vi "LVClass_WavefrontCorrectorSet Get WavefrontCorrectorParameter.vi"(0 "WavefrontCorrectorSet in":refnum<class "WavefrontCorrectorSet.lvclass">, 11 "error in (no error)":errorcluster) -> (4 "WavefrontCorrectorSet out":refnum<class "WavefrontCorrectorSet.lvclass">, 6 "AllCurrentValueSetAndGet":T1[](array[typedef]), 8 "AllCurrentValueGet":T1[](array[typedef]), 15 "error out":errorcluster)   [LabVIEW 2020, in "WavefrontCorrectorSet.lvclass"]
doc: "WavefrontCorrector parameter name getter given its position in the parameters\nlist.\n\n--------------------------------------------------------------------------------\n\n<B>wavefrontcorrector_setIn </B> : WavefrontCorrectorSet object.\n<B>wavefrontcorrector_setOut </B> : WavefrontCorrectorSet object.\n<B>index </B> : Parameter index.\n<B>parameter_name </B> : Parameter name.\n<B>ErrorIn </B> : Error\n<B>ErrorOut </B> : Error\n\n--------------------------------------------------------------------------------"
uses:
  WavefrontCorrectorSet.lvclass
  CameraParametersSetup.ctl
  CameraParameters_Type.ctl
  WavefrontCorrectorSet.lvclass/WavefrontCorrectorSet.ctl
  LVClass_WavefrontCorrectorSet Read AllValueSetAndGet.vi
  LVClass_WavefrontCorrectorSet Read AllValueGet.vi
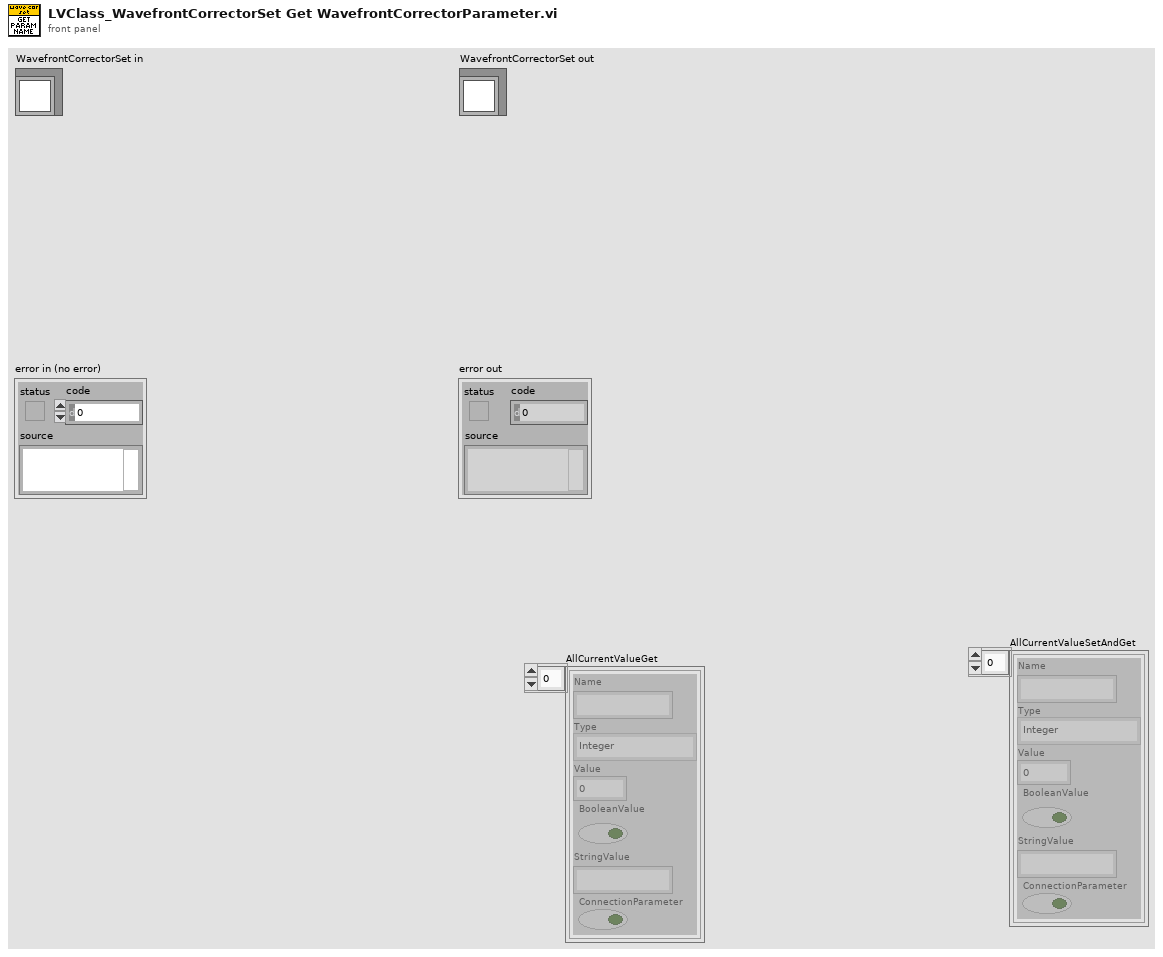
[diagram p1: front panel]
types:
  T1 = typedef "CameraParametersSetup.ctl" = cluster{"Name":string, "Type":T2, "Value":dbl, "BooleanValue":bool, "StringValue":string, "ConnectionParameter":bool}
  T2 = typedef "CameraParameters_Type.ctl" = enum16{"Integer", "Real", "String", "Boolean"}
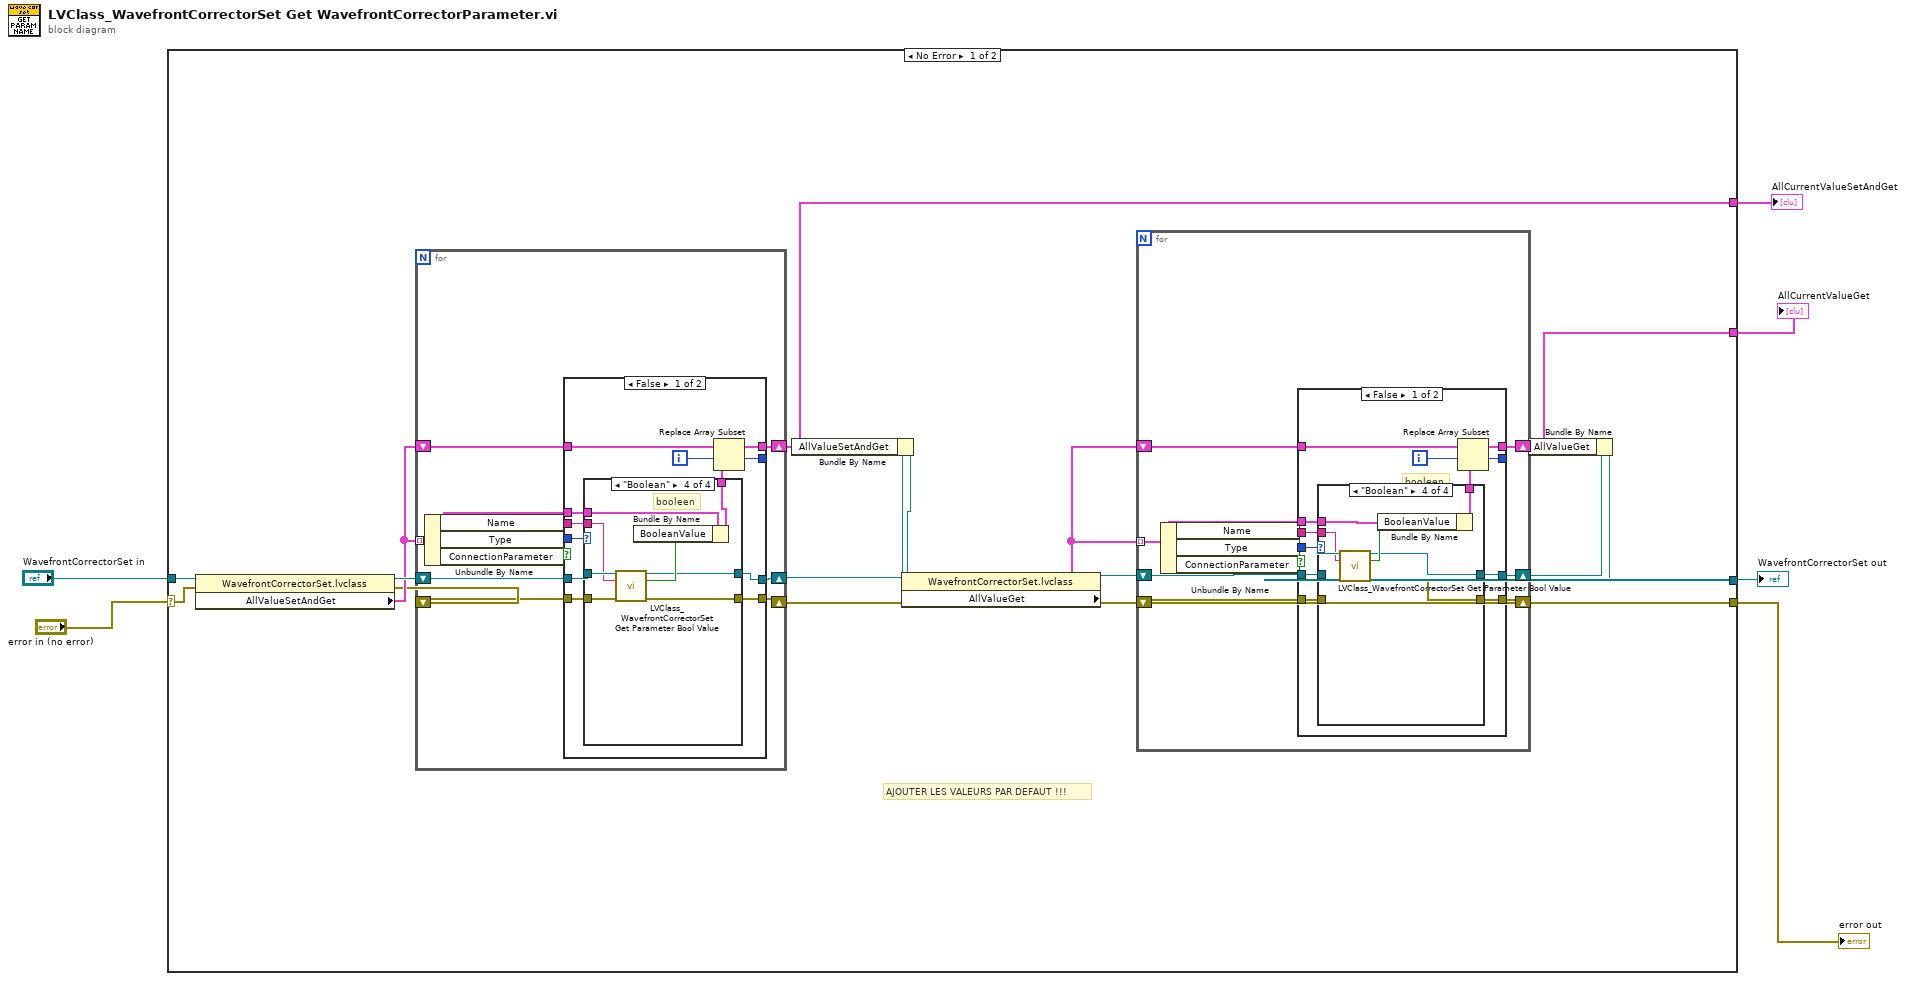
[diagram p0: block diagram]
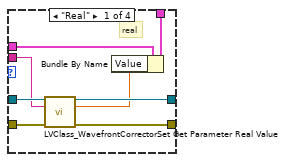
[diagram p2: hidden frame]
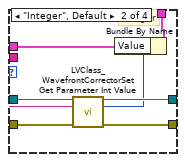
[diagram p3: hidden frame]
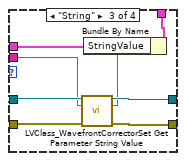
[diagram p4: hidden frame]
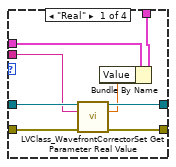
[diagram p6: hidden frame]
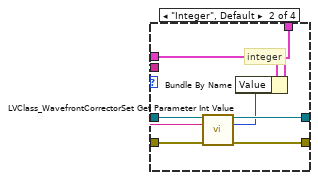
[diagram p7: hidden frame]
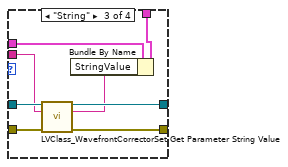
[diagram p8: hidden frame]
diagram:
  n1 = case shown="No Error" "error in (no error)" {
    selector: "error in (no error)" -> [w8 w136]
    tunnel: "WavefrontCorrectorSet in" -> [w11 w137]
    tunnel: [w10 w137] -> w4
    tunnel: [w12 _] -> w2
    tunnel: [w9 w136] -> w3
    tunnel: [w7 _] -> w1
    frame No Error {
      # "AJOUTER LES VALEURS PAR DEFAUT !!!"
      n2 = property class="WavefrontCorrectorSet.lvclass"(reference=w11, error in=w8) -> (reference out=w20:refnum<class "WavefrontCorrectorSet.lvclass">, error out=w18:errorcluster, "AllValueSetAndGet"=w19:T1[])
      n3 = for {
        shift-right: [w89] -> w15
        shift-left: w18 -> [w82]
        shift-right: [w88] -> w21
        shift-left: w20 -> [w83]
        shift-right: [w86] -> w12
        shift-left: w19 -> [w87]
        tunnel: w19 -> [w80] mode=indexing
        i -> [w85]
        n4 = Unbundle By Name(w80) -> ("Name"=w84:string, "Type"=w81:T2, "ConnectionParameter"=w79:bool)
        n5 = case shown="False" w79 {
          tunnel: [w100 w133] -> w89
          tunnel: [w99 w134] -> w88
          tunnel: w87 -> [w98 w135]
          tunnel: [w97 w135] -> w86
          tunnel: w85 -> [w96 _]
          tunnel: w84 -> [w94 _]
          tunnel: w83 -> [w93 w134]
          tunnel: w82 -> [w92 w133]
          tunnel: w81 -> [w91 _]
          tunnel: w80 -> [w90 _]
          frame False {
            n6 = case shown="\"Boolean\"" w91 {
              tunnel: w90 -> [w102 w109 w118 w131]
              tunnel: w94 -> [w106 w114 w120 w128]
              tunnel: [w105 w113 w122 w126] -> w100
              tunnel: w93 -> [w108 w116 w124 w130]
              tunnel: w92 -> [w107 w115 w121 w129]
              tunnel: [w104 w112 w123 w127] -> w99
              tunnel: [w103 w111 w117 w125] -> w95
              frame "Real" {
                n7 = call "LVClass_WavefrontCorrectorSet Get Parameter Real Value.vi"("WavefrontCorrectorSet in"=w108, "parameter_name"=w106, "error in (no error)"=w107) -> ("WavefrontCorrectorSet out"=w104:refnum<class "WavefrontCorrectorSet.lvclass">, "Value"=w101:dbl, "error out"=w105:errorcluster)  [unwired: 10 in]
                n8 = Bundle By Name(cluster=w102, "Value"=w101) -> (w103:T1)
              }
              frame "Integer", Default {
                # "integer"
                n9 = call "LVClass_WavefrontCorrectorSet Get Parameter Int Value.vi"("WavefrontCorrectorSet in"=w116, "parameter_name"=w114, "error in (no error)"=w115) -> ("WavefrontCorrectorSet out"=w112:refnum<class "WavefrontCorrectorSet.lvclass">, "Value"=w110:i32, "error out"=w113:errorcluster)  [unwired: 10 in]
                n10 = Bundle By Name(cluster=w109, "Value"=w110) -> (w111:T1)
              }
              frame "String" {
                n11 = call "LVClass_WavefrontCorrectorSet Get Parameter String Value.vi"("WavefrontCorrectorSet in"=w124, "parameter name"=w120, "error in (no error)"=w121) -> ("WavefrontCorrectorSet out"=w123:refnum<class "WavefrontCorrectorSet.lvclass">, "Value"=w119:string, "error out"=w122:errorcluster)  [unwired: 10 in]
                n12 = Bundle By Name(cluster=w118, "StringValue"=w119) -> (w117:T1)
              }
              frame "Boolean" {
                # "booleen"
                n13 = call "LVClass_WavefrontCorrectorSet Get Parameter Bool Value.vi"("WavefrontCorrectorSet in"=w130, "parameter_name"=w128, "error in (no error)"=w129) -> ("WavefrontCorrectorSet out"=w127:refnum<class "WavefrontCorrectorSet.lvclass">, "Value"=w132:bool, "error out"=w126:errorcluster)  [unwired: 10 in]
                n14 = Bundle By Name(cluster=w131, "BooleanValue"=w132) -> (w125:T1)
              }
            }
            n15 = Replace Array Subset(array=w98, new element=w95, index=w96) -> (w97:T1[])
          }
          frame True {
          }
        }
      }
      n16 = Bundle By Name(cluster=w21, "AllValueSetAndGet"=w12) -> (w16:refnum<class "WavefrontCorrectorSet.lvclass">)
      n17 = property class="WavefrontCorrectorSet.lvclass"(reference=w16, error in=w15) -> (reference out=w17:refnum<class "WavefrontCorrectorSet.lvclass">, error out=w9:errorcluster, "AllValueGet"=w13:T1[])
      n18 = for {
        shift-right: [w32] -> _
        shift-left: w9 -> [w25]
        shift-right: [w31] -> w14
        shift-left: w17 -> [w26]
        shift-right: [w29] -> w7
        shift-left: w13 -> [w30]
        tunnel: w13 -> [w23] mode=indexing
        i -> [w28]
        n19 = Unbundle By Name(w23) -> ("Name"=w27:string, "Type"=w24:T2, "ConnectionParameter"=w22:bool)
        n20 = case shown="False" w22 {
          tunnel: [w43 w76] -> w32
          tunnel: [w42 w77] -> w31
          tunnel: w30 -> [w41 w78]
          tunnel: [w40 w78] -> w29
          tunnel: w28 -> [w39 _]
          tunnel: w27 -> [w37 _]
          tunnel: w26 -> [w36 w77]
          tunnel: w25 -> [w35 w76]
          tunnel: w24 -> [w34 _]
          tunnel: w23 -> [w33 _]
          frame False {
            n21 = case shown="\"Boolean\"" w34 {
              tunnel: w33 -> [w45 w52 w61 w74]
              tunnel: w37 -> [w49 w57 w63 w71]
              tunnel: [w48 w56 w65 w69] -> w43
              tunnel: w36 -> [w51 w59 w67 w73]
              tunnel: w35 -> [w50 w58 w64 w72]
              tunnel: [w47 w55 w66 w70] -> w42
              tunnel: [w46 w54 w60 w68] -> w38
              frame "Real" {
                # "real"
                n22 = call "LVClass_WavefrontCorrectorSet Get Parameter Real Value.vi"("WavefrontCorrectorSet in"=w51, "parameter_name"=w49, "error in (no error)"=w50) -> ("WavefrontCorrectorSet out"=w47:refnum<class "WavefrontCorrectorSet.lvclass">, "Value"=w44:dbl, "error out"=w48:errorcluster)  [unwired: 10 in]
                n23 = Bundle By Name(cluster=w45, "Value"=w44) -> (w46:T1)
              }
              frame "Integer", Default {
                # "integer"
                n24 = call "LVClass_WavefrontCorrectorSet Get Parameter Int Value.vi"("WavefrontCorrectorSet in"=w59, "parameter_name"=w57, "error in (no error)"=w58) -> ("WavefrontCorrectorSet out"=w55:refnum<class "WavefrontCorrectorSet.lvclass">, "Value"=w53:i32, "error out"=w56:errorcluster)  [unwired: 10 in]
                n25 = Bundle By Name(cluster=w52, "Value"=w53) -> (w54:T1)
              }
              frame "String" {
                n26 = call "LVClass_WavefrontCorrectorSet Get Parameter String Value.vi"("WavefrontCorrectorSet in"=w67, "parameter name"=w63, "error in (no error)"=w64) -> ("WavefrontCorrectorSet out"=w66:refnum<class "WavefrontCorrectorSet.lvclass">, "Value"=w62:string, "error out"=w65:errorcluster)  [unwired: 10 in]
                n27 = Bundle By Name(cluster=w61, "StringValue"=w62) -> (w60:T1)
              }
              frame "Boolean" {
                # "booleen"
                n28 = call "LVClass_WavefrontCorrectorSet Get Parameter Bool Value.vi"("WavefrontCorrectorSet in"=w73, "parameter_name"=w71, "error in (no error)"=w72) -> ("WavefrontCorrectorSet out"=w70:refnum<class "WavefrontCorrectorSet.lvclass">, "Value"=w75:bool, "error out"=w69:errorcluster)  [unwired: 10 in]
                n29 = Bundle By Name(cluster=w74, "BooleanValue"=w75) -> (w68:T1)
              }
            }
            n30 = Replace Array Subset(array=w41, new element=w38, index=w39) -> (w40:T1[])
          }
          frame True {
          }
        }
      }
      n31 = Bundle By Name(cluster=w14, "AllValueGet"=w7) -> (w10:refnum<class "WavefrontCorrectorSet.lvclass">)
    }
    frame Error {
    }
  }
  "error out" <- w3
  "WavefrontCorrectorSet out" <- w4
  "AllCurrentValueSetAndGet" <- w2
  "AllCurrentValueGet" <- w1
